vi "Convert Double to String.vi"(8 "error in":errorcluster, 11 "Numeric":dbl) -> (0 "error out":errorcluster, 3 "PGSQL String":string)   [LabVIEW 2019, in "LV-Data.PGSQL.lvclass"]
uses:
  LV-Data.PGSQL.lvclass
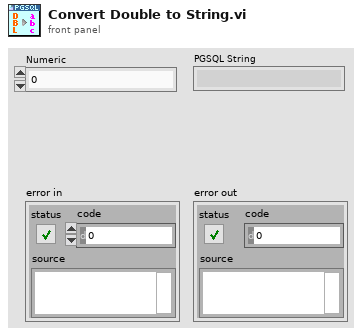
[diagram p1: front panel]
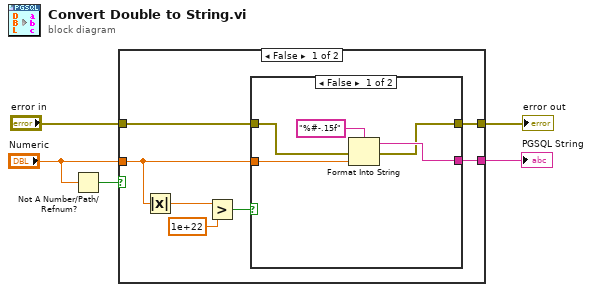
[diagram p0: block diagram]
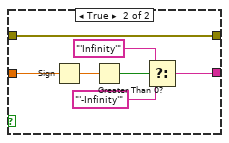
[diagram p2: hidden frame]
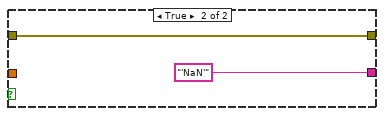
[diagram p3: hidden frame]
diagram:
  n1 = Not A Number/Path/Refnum?(number/path/refnum="Numeric") -> (NaN/Path/Refnum?=w4:bool)
  n2 = case shown="False" w4 {
    tunnel: "Numeric" -> [w8 _]
    tunnel: [w12 "'NaN'"] -> w3
    tunnel: "error in" -> [w7 w25]
    tunnel: [w6 w25] -> w1
    frame False {
      n3 = Absolute Value(x=w8) -> (abs(x)=w10:dbl)
      n4 = Greater?(x=w10, y=1e+22 ("x")) -> (0:w9:bool)
      n5 = case shown="False" w9 {
        tunnel: [w17 w23] -> w12
        tunnel: w8 -> [w15 w20]
        tunnel: w7 -> [w13 w18]
        tunnel: [w14 w18] -> w6
        frame False {
          n6 = Format Into String(format string="%#-.15f", error in=w13, w15) -> (resulting string=w17:string, error out=w14:errorcluster)  [unwired: 1 in]
        }
        frame True {
          n7 = Sign(1:w20) -> (0:w19:dbl)
          n8 = Greater Than 0?(x=w19) -> (x > 0?=w24:bool)
          n9 = Select(t="'Infinity'", s=w24, f="'-Infinity'") -> (s? t:f=w23:string)
        }
      }
    }
    frame True {
    }
  }
  "PGSQL String" <- w3
  "error out" <- w1
